vi "get_elements_in_queue.vi"(11 "on-board buffer in":T1) -> (2 "no. elements":u32)   [LabVIEW 2010, in "OnBoardBuffer.lvlib"]
uses:
  OnBoardBuffer.lvlib
  OnBoardBuffer.ctl
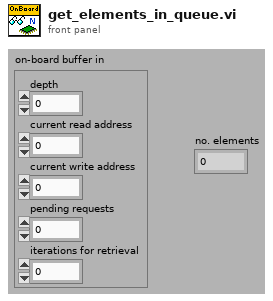
[diagram p1: front panel]
types:
  T1 = typedef "OnBoardBuffer.lvlib/OnBoardBuffer.ctl" = cluster{"depth":u32, "current read address":u32, "current write address":u32, "pending requests":u32, "iterations for retrieval":u32}
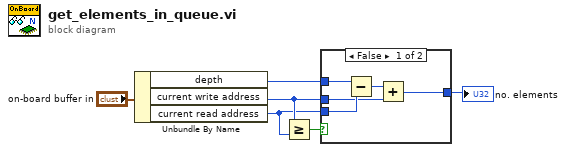
[diagram p0: block diagram]
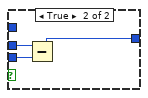
[diagram p2: hidden frame]
diagram:
  n1 = Unbundle By Name("on-board buffer in") -> ("depth"=w6:u32, "current write address"=w5:u32, "current read address"=w4:u32)
  n2 = Greater Or Equal?(x=w5, y=w4) -> (x >= y?=w3:bool)
  n3 = case shown="False" w3 {
    tunnel: w6 -> [w11 _]
    tunnel: w4 -> [w10 w14]
    tunnel: w5 -> [w8 w13]
    tunnel: [w7 w12] -> w1
    frame False {
      n4 = Subtract(x=w11, y=w10) -> (x-y=w9:u32)
      n5 = Add(x=w9, y=w8) -> (x+y=w7:u32)
    }
    frame True {
      n6 = Subtract(x=w13, y=w14) -> (x-y=w12:u32)
    }
  }
  "no. elements" <- w1
